vi "Fitra per tabella.vi"(10 "TAB":i32, 11 "dati in":string[][](array[string])) -> (3 "dati out":string[][](array[string]))   [LabVIEW 2019]
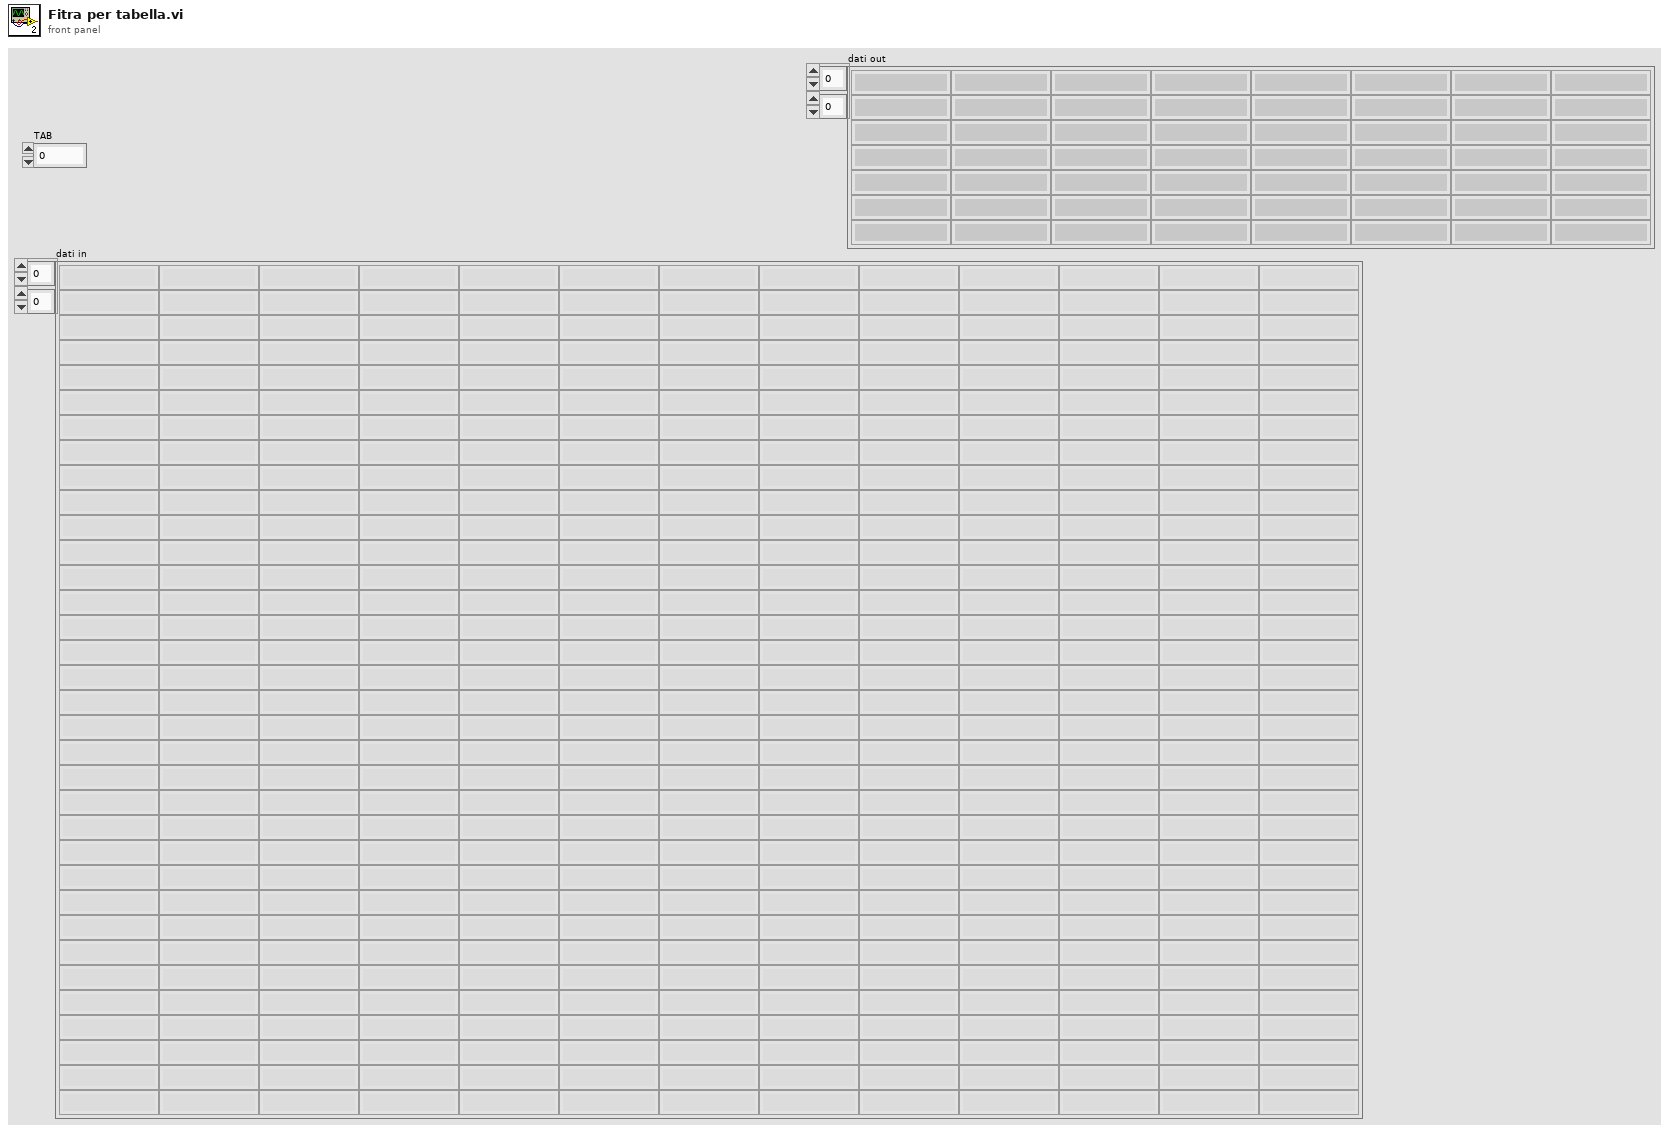
[diagram p1: front panel]
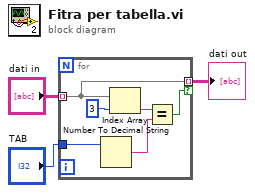
[diagram p0: block diagram]
diagram:
  n1 = for {
    tunnel: "dati in" -> [w5] mode=indexing
    tunnel: "TAB" -> [w8]
    tunnel: [w5] -> w3 mode=indexing if=w4
    n2 = Number To Decimal String(number=w8) -> (decimal integer string=w6:string)  [unwired: 1 in]
    n3 = Index Array(array=w5, index=3) -> (element=w7:string)
    n4 = Equal?(x=w7, y=w6) -> (x = y?=w4:bool)
  }
  "dati out" <- w3
